vi "3D-ReleaseROIStringtoArray.vi"(11 "ROI Information":string[](array[string])=["A:{446.000;118.000;566.000;162.000;0.000}"]) -> (0 "B ROI Param":dbl[](array[numeric]), 1 "B_label":string, 2 "A_label":string, 3 "A ROI Param":dbl[](array[numeric]), 4 "B ROI Param":string[](array[string]), 5 "A ROI Param":string[](array[string]))   [LabVIEW 2015]
panel:
  out "结果字符串 2":string
  out "结果字符串":string
  out "元素":string
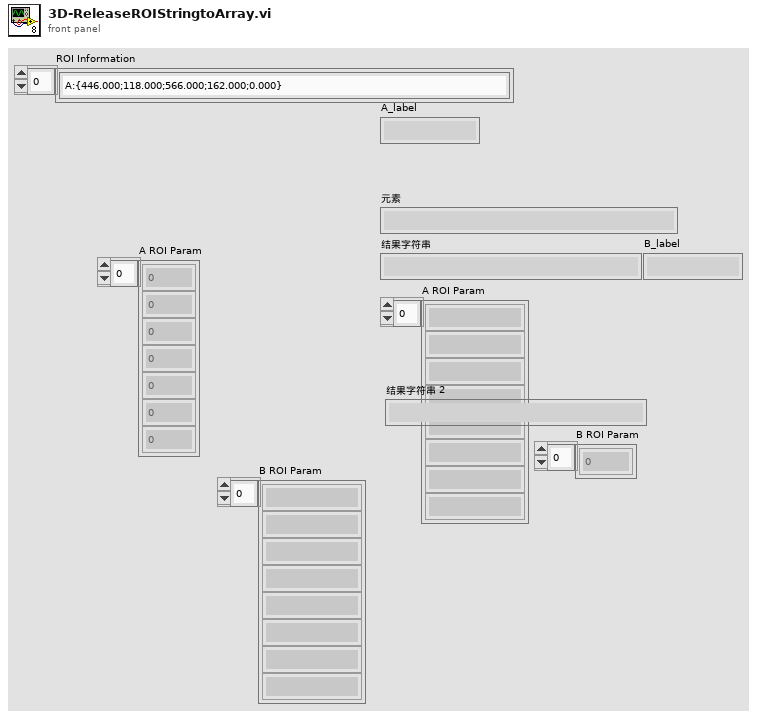
[diagram p1: front panel]
types:
  T1 = typedef "IMAQ Rectangle" = cluster{"Left":i32, "Top":i32, "Right":i32, "Bottom":i32, "Rotation":dbl}
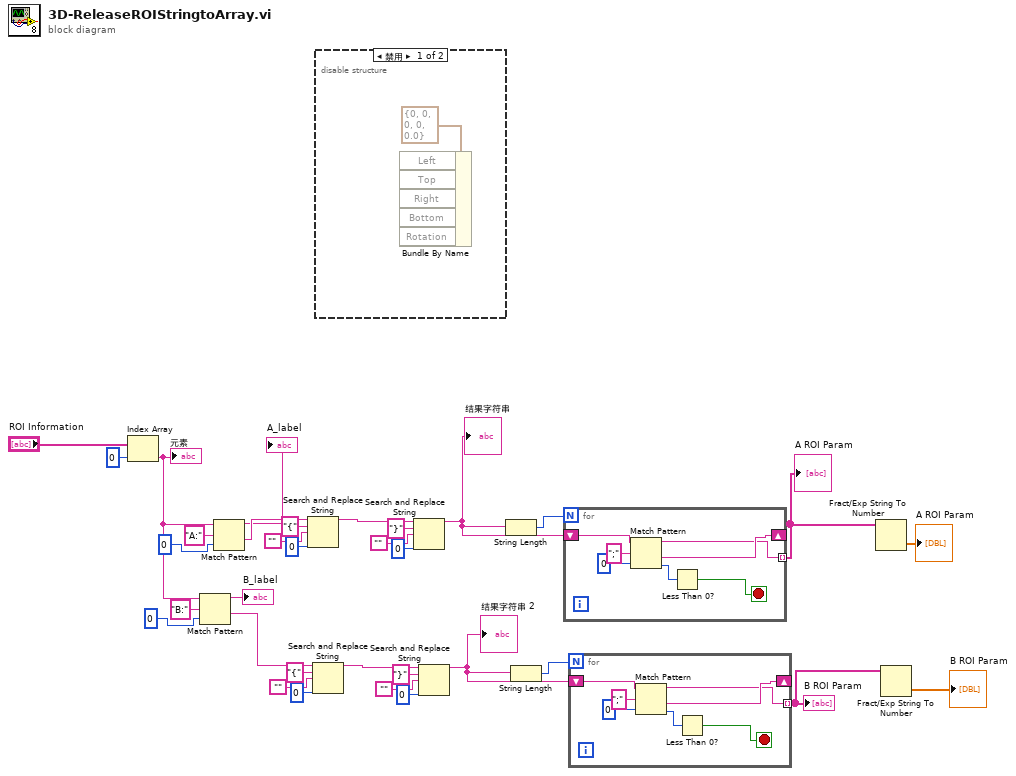
[diagram p0: block diagram]
diagram:
  n1 = Index Array(array="ROI Information", index=0 ("索引")) -> (element=w27:string)
  "元素" <- w27
  n2 = Match Pattern(string=w27, regular expression="B:" ("正则表达式"), offset (0)=0 ("偏移量(0)")) -> (before substring=→"B_label":string, after substring=w4:string)  [unwired: 2 out]
  n3 = Match Pattern(string=w27, regular expression="A:" ("正则表达式"), offset (0)=0 ("偏移量(0)")) -> (before substring=→"A_label":string, after substring=w26:string)  [unwired: 2 out]
  n4 = Search and Replace String(input string=w26, search string="{" ("搜索字符串"), replace string="", offset=0 ("偏移量(0)")) -> (result string=w19:string)  [unwired: 4 in, 3 out]
  n5 = Search and Replace String(input string=w4, search string="{" ("搜索字符串"), replace string="", offset=0 ("偏移量(0)")) -> (result string=w11:string)  [unwired: 4 in, 3 out]
  n6 = disable-structure shown="禁用" {
    frame Disabled {
      n7 = Bundle By Name(cluster=T1 {"Left"=0, "Top"=0, "Right"=0, "Bottom"=0, "Rotation"=0.0} ("Rectangle")) -> ()  [unwired: 5 in, 1 out]
    }
    frame Enabled {
    }
  }
  n8 = Search and Replace String(input string=w19, search string="}" ("搜索字符串"), replace string="", offset=0 ("偏移量(0)")) -> (result string=w17:string)  [unwired: 4 in, 3 out]
  "结果字符串" <- w17
  n9 = Search and Replace String(input string=w11, search string="}" ("搜索字符串"), replace string="", offset=0 ("偏移量(0)")) -> (result string=w13:string)  [unwired: 4 in, 3 out]
  "结果字符串 2" <- w13
  n10 = String Length(string=w17) -> (length=w18:i32)
  n11 = String Length(string=w13) -> (length=w12:i32)
  n12 = for {
    N: w18 -> [_]
    shift-right: [w36] -> _
    shift-left: w17 -> [w41]
    tunnel: [w35] -> w16 mode=indexing
    stop <- w37 stop-if-true
    n13 = Match Pattern(string=w41, regular expression=";" ("正则表达式"), offset (0)=0 ("偏移量(0)")) -> (before substring=w35:string, after substring=w36:string, offset past match=w38:i32)  [unwired: 1 out]
    n14 = Less Than 0?(x=w38) -> (x < 0?=w37:bool)
  }
  "A ROI Param" <- w16
  n15 = for {
    N: w12 -> [_]
    shift-right: [w43] -> _
    shift-left: w13 -> [w48]
    tunnel: [w42] -> w14 mode=indexing
    stop <- w44 stop-if-true
    n16 = Match Pattern(string=w48, regular expression=";" ("正则表达式"), offset (0)=0 ("偏移量(0)")) -> (before substring=w42:string, after substring=w43:string, offset past match=w45:i32)  [unwired: 1 out]
    n17 = Less Than 0?(x=w45) -> (x < 0?=w44:bool)
  }
  "B ROI Param" <- w14
  n18 = Fract/Exp String To Number(string=w16) -> (number=→"A ROI Param":dbl[])  [unwired: 3 in, 1 out]
  n19 = Fract/Exp String To Number(string=w14) -> (number=→"B ROI Param":dbl[])  [unwired: 3 in, 1 out]
